vi "mainlooproutine.vi"(10 "Loop Cluster":T4, 11 "Device Cluster":T3={"K2400 1"="", "K2400_1"=FALSE, "K2400 2"="", "K2400_2"=FALSE, "Lockin1"="", "Lockin1 present"=FALSE, "Lockin2"="", "Lockin2 present"=FALSE, "TIC"="", "Tcontrol"="OFF", "DMM1"="", "DMM1"=FALSE, "DMM2"="", "DMM2"=FALSE, "DAC"="", "DAC present"=FALSE, "DAC number"=0, "Bfield query"=FALSE, "Wvlen query"=FALSE, "ITC signal"={"ITC"=0, "Signal"=enum."Sensor 1"}}) -> ()   [LabVIEW 2011]
uses:
  Kelvinox drivers/ITCAPPS - Copie.LLB/ITCSignal.ctl
  Kelvinox drivers/ITCAPPS - Copie.LLB/ITCSignals.ctl
panel:
  in  "Instrument array":string[](array[string])
  in  "Array In":dbl[][](array[numeric])
  out "Current sweep":dbl
  out "ITC ref":T1={"ITC"=0, "Signal"=enum."Sensor 3"}
  in  "Cancel run":bool
  out "DAC number":u8
  out "DAC":refnum<visa-resource-name>
  out "K2400 2":refnum<visa-resource-name>
  out "Lockin1":refnum<visa-resource-name>
  out "K2400 1":refnum<visa-resource-name>
  in  "Sweep Instrument":string(combo)
  in  "Conversion Factor Fix\n1 V = ??":dbl=1.0
  in  "Fix Instrument":string(combo)
  in  "Conversion Factor Sweep\n1 V = ??":dbl=1.0
  in  "Step Delay (ms)":dbl=1000.0
  in  "Rate [T/min]":dbl=-1.0 min=-200.0 max=200.0
  out "Total Progress":dbl(slide) scale=0.0..1.0
  # "Magnetic Field"
  # "Wavelength"
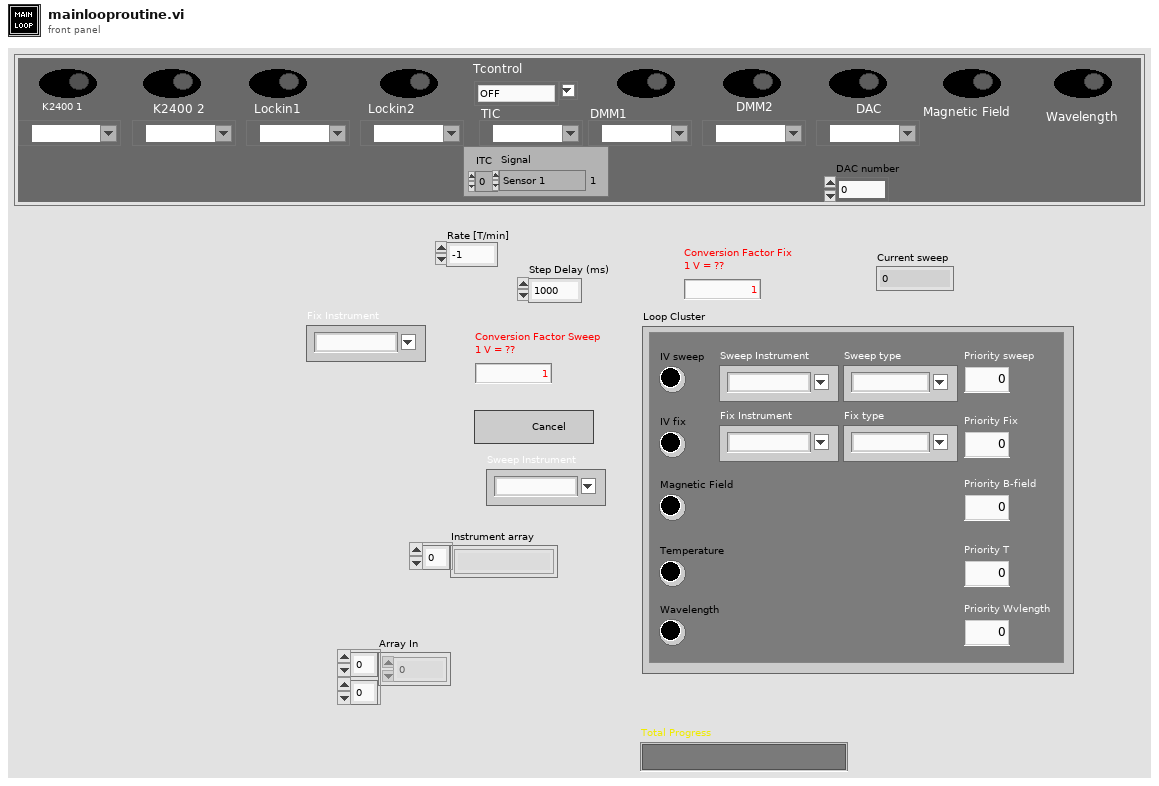
[diagram p1: front panel]
types:
  T1 = typedef "ITCSignal.ctl" = cluster{"ITC":u16, "Signal":T2}
  T2 = typedef "ITCSignals.ctl" = enum16{"Setpoint", "Sensor 1", "Sensor 2", "Sensor 3", "Needle Valve %", "Heater %"}
  T3 = cluster{"K2400 1":refnum<visa-resource-name>, "K2400_1":bool, "K2400 2":refnum<visa-resource-name>, "K2400_2":bool, "Lockin1":refnum<visa-resource-name>, "Lockin1 present":bool, "Lockin2":refnum<visa-resource-name>, "Lockin2 present":bool, "TIC":refnum<visa-resource-name>, "Tcontrol":string, "DMM1":refnum<visa-resource-name>, "DMM1":bool, "DMM2":refnum<visa-resource-name>, "DMM2":bool, "DAC":refnum<visa-resource-name>, "DAC present":bool, "DAC number":u8, "Bfield query":bool, "Wvlen query":bool, "ITC signal":T1}
  T4 = cluster{"Sweep Instrument":string, "Sweep type":string, "Fix Instrument":string, "Fix type":string, "IV sweep":bool, "IV fix":bool, "Magnetic Field":bool, "Temperature":bool, "Wavelength":bool, "Priority sweep":dbl, "Priority Fix":dbl, "Priority B-field":dbl, "Priority T":dbl, "Priority Wvlength":dbl}
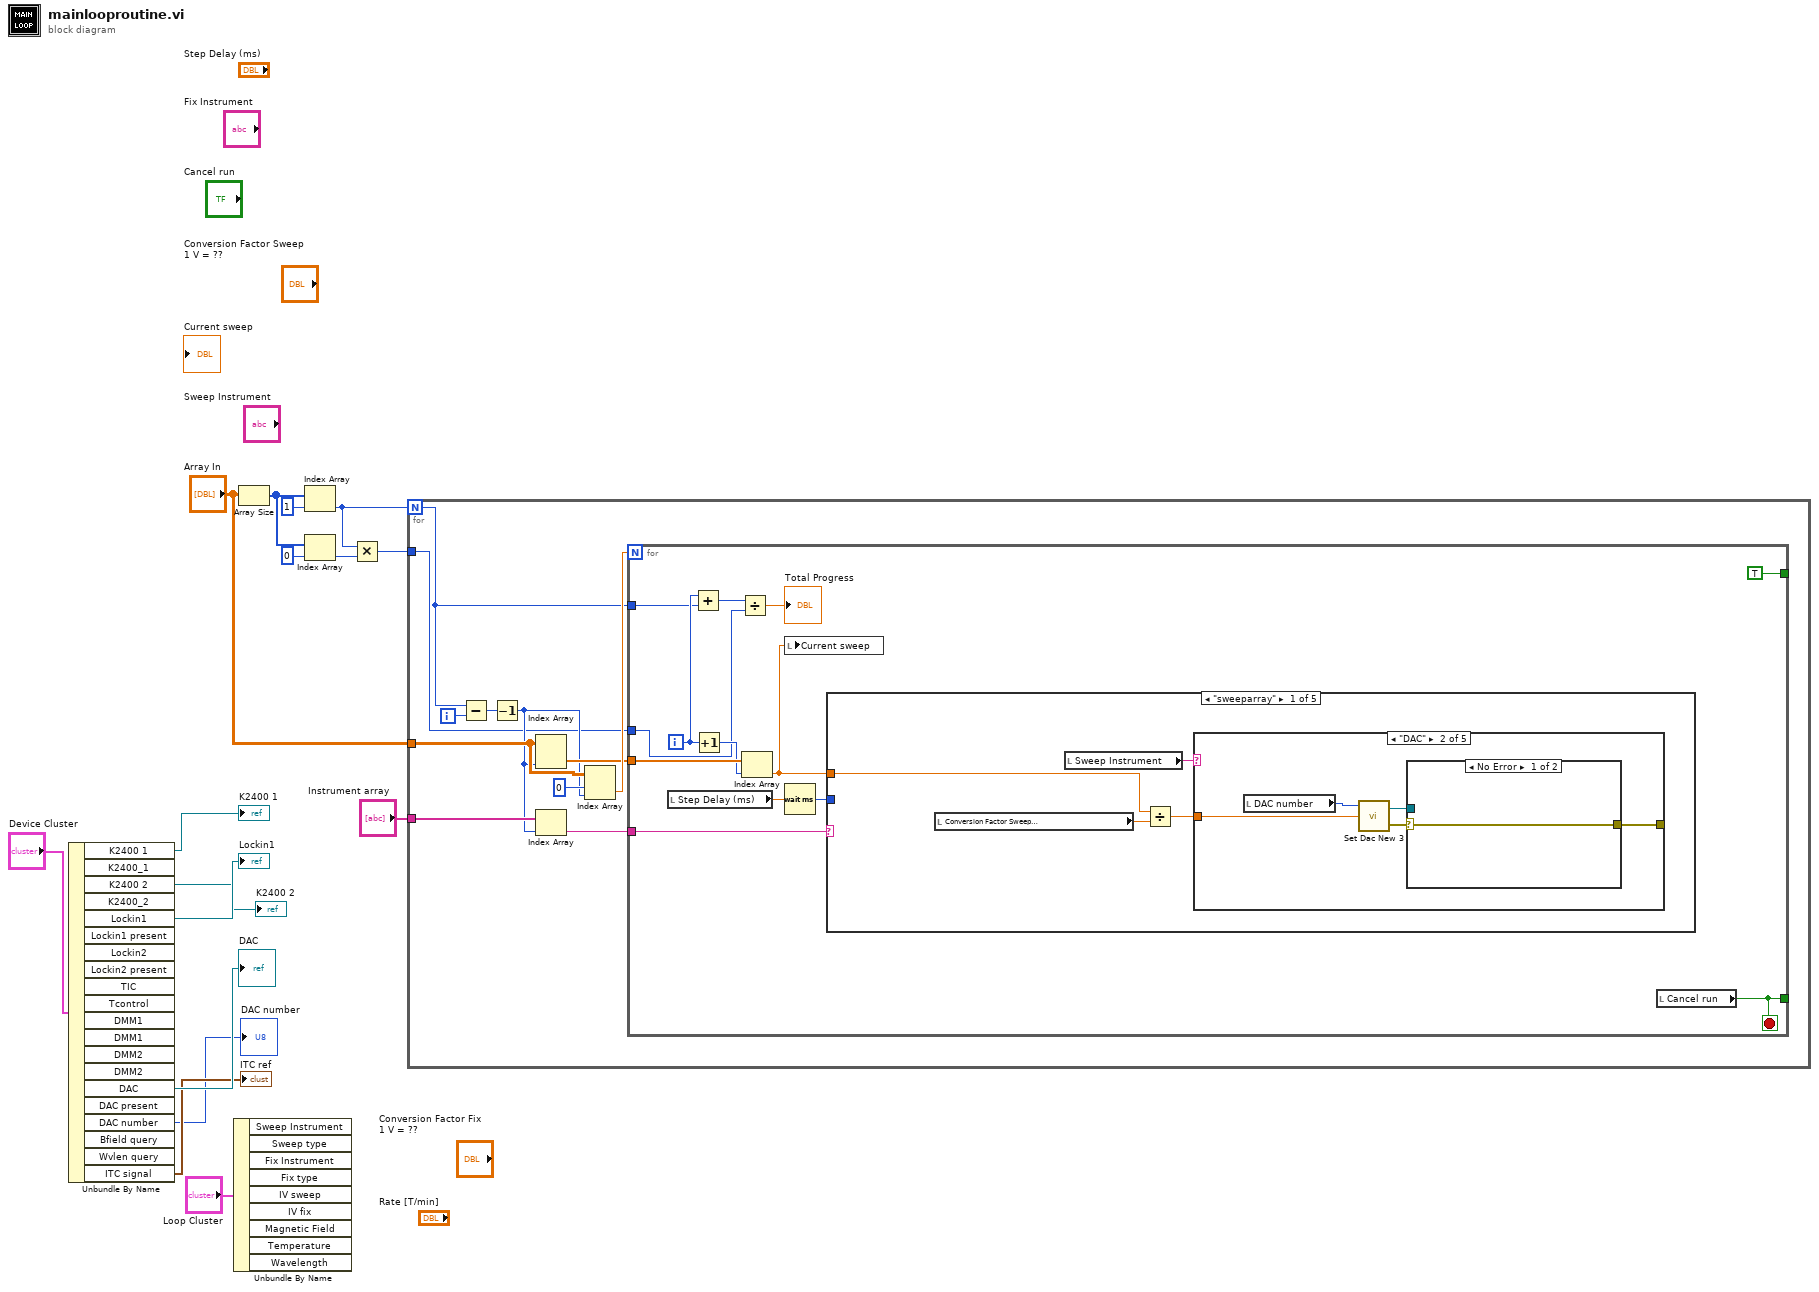
[diagram p0: block diagram]
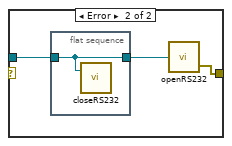
[diagram p3: hidden frame]
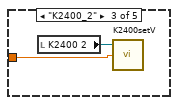
[diagram p4: hidden frame]
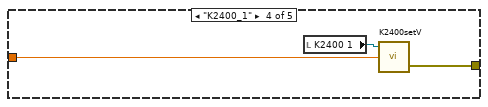
[diagram p5: hidden frame]
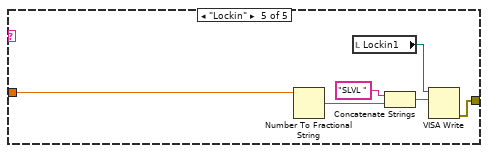
[diagram p6: hidden frame]
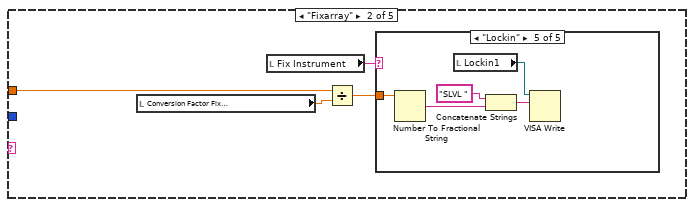
[diagram p7: hidden frame]
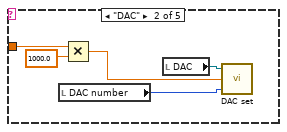
[diagram p9: hidden frame]
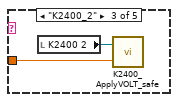
[diagram p10: hidden frame]
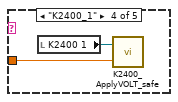
[diagram p11: hidden frame]
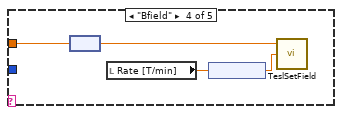
[diagram p13: hidden frame]
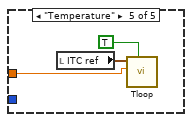
[diagram p14: hidden frame]
diagram:
  n1 = Unbundle By Name("Device Cluster") -> ("K2400 1"=→"K2400 1":refnum<visa-resource-name>, "K2400 2"=→"K2400 2":refnum<visa-resource-name>, "Lockin1"=→"Lockin1":refnum<visa-resource-name>, "DAC"=→"DAC":refnum<visa-resource-name>, "DAC number"=→"DAC number":u8, "ITC signal"=→"ITC ref":T1)  [unwired: 14 out]
  n2 = Unbundle By Name("Loop Cluster") -> ()  [unwired: 9 out]
  n3 = Array Size(array="Array In") -> (size(s)=w12:i32[])
  n4 = Index Array(array=w12, index=1) -> (element=w9:i32)
  n5 = Index Array(array=w12, index=0) -> (element=w10:i32)
  n6 = Multiply(x=w9, y=w10) -> (x*y=w8:i32)
  n7 = for {
    N: w9 -> [w18]
    tunnel: "Array In" -> [w23]
    tunnel: "Instrument array" -> [w21]
    tunnel: w8 -> [w17]
    i -> [w26]
    n8 = Subtract(x=w18, y=w26) -> (x-y=w25:i32)
    n9 = Decrement(x=w25) -> (x-1=w20:i32)
    n10 = Index Array(array=w23, index (col)=w20) -> (element=w22:dbl[])  [unwired: 1 in]
    n11 = Index Array(array=w21, index=w20) -> (element=w19:string)
    n12 = Index Array(array=w23, index (row)=0, index (col)=w20) -> (element=w24:dbl)
    n13 = for {
      N: w24 -> [_]
      tunnel: [TRUE ("stopsignal")] -> _
      tunnel: w22 -> [w39]
      tunnel: w19 -> [w38]
      tunnel: w17 -> [w36]
      tunnel: w18 -> [w33]
      tunnel: [w31] -> _
      i -> [w34]
      stop <- w31 stop-if-true
      n14 = local read "Step Delay (ms)"() -> (w29:dbl)
      n15 = Add(x=w34, y=w33) -> (x+y=w32:i32)
      n16 = Increment(x=w34) -> (x+1=w37:i32)
      n17 = Divide(x=w32, y=w36) -> (x/y=→"Total Progress":dbl)
      n18 = Index Array(array=w39, index=w37) -> (element=w30:dbl)
      n19 = local write "Current sweep"(w30) -> ()
      n20 = Wait (ms)(milliseconds to wait=w29) -> (millisecond timer value=w28:u32)
      n21 = case shown="\"sweeparray\"" w38 {
        tunnel: w30 -> [w43 w68 _ w85 w89]
        tunnel: w28 -> [_ _ _ _ _]
        frame "sweeparray" {
          n22 = local read "Conversion Factor Sweep\n1 V = ??"() -> (w44:dbl)
          n23 = local read "Sweep Instrument"() -> (w41:string)
          n24 = Divide(x=w43, y=w44) -> (x/y=w42:dbl)
          n25 = case shown="\"DAC\"" w41 {
            tunnel: w42 -> [_ w48 w56 w59 w62]
            tunnel: [_ w45 _ w57 w60] -> _
            frame Default {
            }
            frame "DAC" {
              n26 = local read "DAC number"() -> (w49:u8)
              n27 = call "Set Dac New 3.vi"("DATA (V)"=w48, "DAC nr"=w49) -> ("error out"=w47:errorcluster, "VISA resource name OUT"=w46:refnum<visa-resource-name>)  [unwired: 1 in]
              n28 = case shown="No Error" w47 {
                selector: w47 -> [w50 _]
                tunnel: w46 -> [_ w53]
                tunnel: [w50 w51] -> w45
                frame No Error {
                }
                frame Error {
                  n29 = flat-sequence {
                    tunnel: w53 -> [w54]
                    tunnel: [w54] -> w52
                    frame #0 {
                      n30 = call "closeRS232.vi"("VISA resource name"=w54) -> ()  [unwired: 2 in]
                    }
                  }
                  n31 = call "openRS232.vi"("com"=w52) -> ("error out"=w51:errorcluster)  [unwired: 1 out]
                }
              }
            }
            frame "K2400_2" {
              n32 = local read "K2400 2"() -> (w55:refnum<visa-resource-name>)
              n33 = call "K2400setV.vi"("Voltage target [V]"=w56, "VISA Resource Name"=w55) -> ()  [unwired: 1 in, 2 out]
            }
            frame "K2400_1" {
              n34 = local read "K2400 1"() -> (w58:refnum<visa-resource-name>)
              n35 = call "K2400setV.vi"("Voltage target [V]"=w59, "VISA Resource Name"=w58) -> ("error out"=w57:errorcluster)  [unwired: 1 in, 1 out]
            }
            frame "Lockin" {
              n36 = Number To Fractional String(number=w62) -> (F-format string=w65:string)  [unwired: 3 out]
              n37 = local read "Lockin1"() -> (w61:refnum<visa-resource-name>)
              n38 = Concatenate Strings("SLVL " ("chaîne"), w65) -> (w63:string)
              n39 = VISA Write(VISA resource name=w61, write buffer=w63) -> (error out=w60:errorcluster)  [unwired: 1 in, 2 out]
            }
          }
        }
        frame "Fixarray" {
          n40 = local read "Conversion Factor Fix\n1 V = ??"() -> (w69:dbl)
          n41 = local read "Fix Instrument"() -> (w66:string)
          n42 = Divide(x=w68, y=w69) -> (x/y=w67:dbl)
          n43 = case shown="\"Lockin\"" w66 {
            tunnel: w67 -> [_ w72 w76 w78 w80]
            frame Default {
            }
            frame "DAC" {
              n44 = local read "DAC number"() -> (w70:u8)
              n45 = Multiply(x=w72, y=1000.0) -> (x*y=w74:dbl)
              n46 = local read "DAC"() -> (w71:refnum<visa-resource-name>)
              n47 = call "DAC set.vi"("DAC number"=w70, "DAC set [mV]"=w74, "DAC COM port"=w71) -> ()  [unwired: 1 out]
            }
            frame "K2400_2" {
              n48 = local read "K2400 2"() -> (w75:refnum<visa-resource-name>)
              n49 = call "K2400_ApplyVOLT_safe.vi"("Voltage target [V]"=w76, "VISA Resource Name"=w75) -> ()  [unwired: 1 in]
            }
            frame "K2400_1" {
              n50 = local read "K2400 1"() -> (w77:refnum<visa-resource-name>)
              n51 = call "K2400_ApplyVOLT_safe.vi"("Voltage target [V]"=w78, "VISA Resource Name"=w77) -> ()  [unwired: 1 in]
            }
            frame "Lockin" {
              n52 = Number To Fractional String(number=w80) -> (F-format string=w83:string)  [unwired: 3 out]
              n53 = local read "Lockin1"() -> (w79:refnum<visa-resource-name>)
              n54 = Concatenate Strings("SLVL " ("chaîne"), w83) -> (w81:string)
              n55 = VISA Write(VISA resource name=w79, write buffer=w81) -> ()  [unwired: 1 in, 3 out]
            }
          }
        }
        frame Default {
        }
        frame "Bfield" {
          n56 = node(w85) -> (w84:dbl[unit])
          n57 = local read "Rate [T/min]"() -> (w86:dbl)
          n58 = node(w86) -> (w87:dbl[unit])
          n59 = call "TeslSetField.vi"("Sweep rate"=w87, "Field required:"=w84) -> ()  [unwired: 2 in, 2 out]
        }
        frame "Temperature" {
          n60 = local read "ITC ref"() -> (w90:T1)
          n61 = call "Tloop.vi"("ITCSignal"=w90, "T target [K]"=w89, "Regulate ?"=TRUE) -> ()  [unwired: 2 in, 2 out]
        }
      }
      n62 = local read "Cancel run"() -> (w31:bool)
    }
  }
